vi "array2Mem_32bit_1to22_pipe.vi"(6 "Address (Max = 255)":u8=24, 10 "ziyi_in":T1=[0.0, 0.0, 0.0, 0.0, 0.0, 0.0, 0.0, 0.0, 0.0, 0.0, 0.0, 0.0, 0.0, 0.0, 0.0, 0.0, 0.0, 0.0, 0.0, 0.0, 0.0, 0.0]) -> ()   [LabVIEW 2017]
uses:
  ziyi_pipe_N22.ctl
  x_qp_scalar.ctl
  typeDefs/QP_mem_type.ctl
  <vilib>/rvi/DataTransferAndStorage/Container/Common/niFpgaContainerExecOnDevCompGetState.vi
  <vilib>/rvi/Emulation/niFpgaEmulationIsFPGAContextNoSignature.vi
  <vilib>/rvi/DataTransferAndStorage/Container/Common/niFpgaContainerGetUniqueNameForEmu.vi
  <vilib>/rvi/Emulation/niFpgaProcessEmulError.vi
  <vilib>/rvi/Emulation/niFpgaSctlEmulationGetInTimedLoop.vi
  <vilib>/rvi/errors/nirviReportUnexpectedCaseInternalError (U32).vi
  <vilib>/rvi/Memory/Memory_Emulation/niFpgaMemoryEmulationCacheClearOnFirstRun.vi
  <vilib>/rvi/Memory/Memory_Emulation/nirvimemoryEmulationManagerCache_MakeExclusive.vi
  <vilib>/rvi/Memory/Memory_Emulation/niFpgaMemoryEmulationValidateCache.vi
  <vilib>/rvi/Memory/Memory_Emulation/nirvimemoryEmulationManagerCache_InsertValue.vi
  <vilib>/Utility/error.llb/Clear Errors.vi
  <vilib>/rvi/Memory/Memory_Emulation/nirvimemoryEmulationManagerCache_ReleaseExclusive.vi
  <vilib>/rvi/Memory/Memory_Emulation/nirvimemoryEmulationManagerCache_GetValue.vi
  <vilib>/rvi/Memory/Memory_Emulation/nirvimemoryEmulationManagerCache_SetValue.vi
  <vilib>/rvi/Emulation/niFpgaSctlEmulationResourceMgr.vi
  <vilib>/rvi/DataTransferAndStorage/Container/XNode/niFpgaContainer.xnode
  <vilib>/rvi/Memory/Memory_Emulation/niFpgaMemoryEmulationRefIn.vi
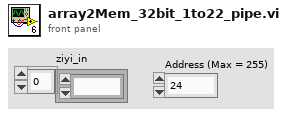
[diagram p1: front panel]
types:
  T1 = typedef "ziyi_pipe_N22.ctl" = T2[]
  T2 = typedef "x_qp_scalar.ctl" = fxp<+/-,32,6>
  T3 = typedef "QP_mem_type.ctl" = refnum<k21>
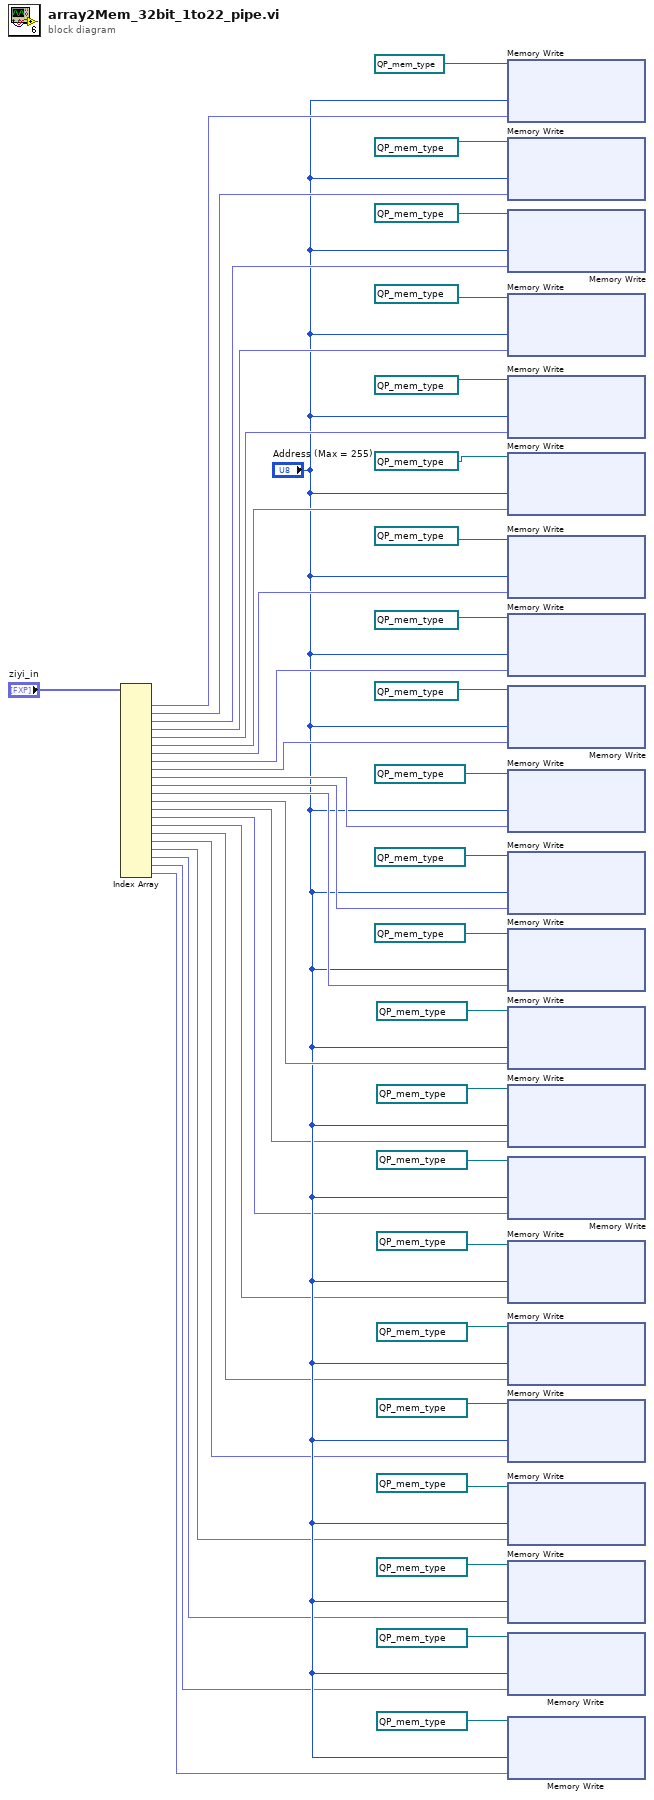
[diagram p0: block diagram]
diagram:
  n1 = Index Array(array="ziyi_in") -> (element #1=w46:T2, element #2=w45:T2, element #3=w44:T2, element #4=w43:T2, element #5=w42:T2, element #6=w41:T2, element #7=w40:T2, element #8=w39:T2, element #9=w38:T2, element #10=w37:T2, element #11=w36:T2, element #12=w23:T2, element #13=w12:T2, element #14=w10:T2, element #15=w9:T2, element #16=w8:T2, element #17=w7:T2, element #18=w6:T2, element #19=w5:T2, element #20=w4:T2, element #21=w3:T2, element #22=w2:T2)  [unwired: 22 in]
  n2 = xnode ("Memory Write")("Address"="Address (Max = 255)", "Data"=w46, "Memory In"=T3 "Memory") -> ()  [unwired: 1 out]
  n3 = xnode ("Memory Write")("Address"="Address (Max = 255)", "Data"=w45, "Memory In"=T3 "Memory 2") -> ()  [unwired: 1 out]
  n4 = xnode ("Memory Write")("Address"="Address (Max = 255)", "Data"=w44, "Memory In"=T3 "Memory 3") -> ()  [unwired: 1 out]
  n5 = xnode ("Memory Write")("Address"="Address (Max = 255)", "Data"=w43, "Memory In"=T3 "Memory 4") -> ()  [unwired: 1 out]
  n6 = xnode ("Memory Write")("Address"="Address (Max = 255)", "Data"=w42, "Memory In"=T3 "Memory 5") -> ()  [unwired: 1 out]
  n7 = xnode ("Memory Write")("Address"="Address (Max = 255)", "Data"=w41, "Memory In"=T3 "Memory 6") -> ()  [unwired: 1 out]
  n8 = xnode ("Memory Write")("Address"="Address (Max = 255)", "Data"=w40, "Memory In"=T3 "Memory 7") -> ()  [unwired: 1 out]
  n9 = xnode ("Memory Write")("Address"="Address (Max = 255)", "Data"=w39, "Memory In"=T3 "Memory 8") -> ()  [unwired: 1 out]
  n10 = xnode ("Memory Write")("Address"="Address (Max = 255)", "Data"=w38, "Memory In"=T3 "Memory 9") -> ()  [unwired: 1 out]
  n11 = xnode ("Memory Write")("Address"="Address (Max = 255)", "Data"=w37, "Memory In"=T3 "Memory 10") -> ()  [unwired: 1 out]
  n12 = xnode ("Memory Write")("Address"="Address (Max = 255)", "Data"=w36, "Memory In"=T3 "Memory 11") -> ()  [unwired: 1 out]
  n13 = xnode ("Memory Write")("Address"="Address (Max = 255)", "Data"=w23, "Memory In"=T3 "Memory 12") -> ()  [unwired: 1 out]
  n14 = xnode ("Memory Write")("Address"="Address (Max = 255)", "Data"=w12, "Memory In"=T3 "Memory 13") -> ()  [unwired: 1 out]
  n15 = xnode ("Memory Write")("Address"="Address (Max = 255)", "Data"=w10, "Memory In"=T3 "Memory 14") -> ()  [unwired: 1 out]
  n16 = xnode ("Memory Write")("Address"="Address (Max = 255)", "Data"=w9, "Memory In"=T3 "Memory 15") -> ()  [unwired: 1 out]
  n17 = xnode ("Memory Write")("Address"="Address (Max = 255)", "Data"=w8, "Memory In"=T3 "Memory 16") -> ()  [unwired: 1 out]
  n18 = xnode ("Memory Write")("Address"="Address (Max = 255)", "Data"=w7, "Memory In"=T3 "Memory 17") -> ()  [unwired: 1 out]
  n19 = xnode ("Memory Write")("Address"="Address (Max = 255)", "Data"=w6, "Memory In"=T3 "Memory 18") -> ()  [unwired: 1 out]
  n20 = xnode ("Memory Write")("Address"="Address (Max = 255)", "Data"=w5, "Memory In"=T3 "Memory 19") -> ()  [unwired: 1 out]
  n21 = xnode ("Memory Write")("Address"="Address (Max = 255)", "Data"=w4, "Memory In"=T3 "Memory 20") -> ()  [unwired: 1 out]
  n22 = xnode ("Memory Write")("Address"="Address (Max = 255)", "Data"=w3, "Memory In"=T3 "Memory 21") -> ()  [unwired: 1 out]
  n23 = xnode ("Memory Write")("Address"="Address (Max = 255)", "Data"=w2, "Memory In"=T3 "Memory 22") -> ()  [unwired: 1 out]
